vi "COM_MA filter.vi"(6 "Fs":dbl, 8 "Error In":errorcluster, 10 "Data In":dbl[](array[numeric])) -> (0 "Error Out":errorcluster, 2 "Data Out":dbl[](array[numeric]))   [LabVIEW 2017, in "AppPlugins.lvlib" / "EraPlugin.lvclass"]
uses:
  EraPlugin.lvclass
  <vilib>/Analysis/4window.llb/windowTd.ctl
  <vilib>/Analysis/3filter.llb/FIR Filter (DBL).vi
  <vilib>/Analysis/4window.llb/Symmetric Window (DBL).vi
  <vilib>/Analysis/NI_AALPro.lvlib
  <vilib>/Analysis/NI_AALBase.lvlib
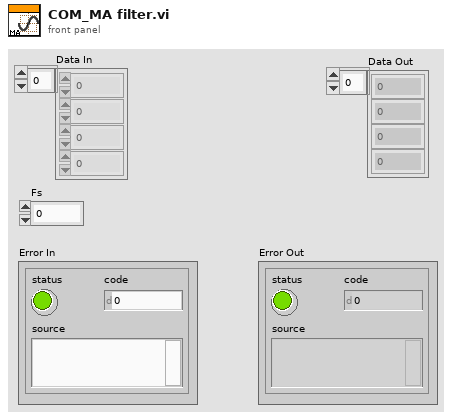
[diagram p1: front panel]
types:
  T1 = typedef "NI_AALPro.lvlib/windowTd.ctl" = u32
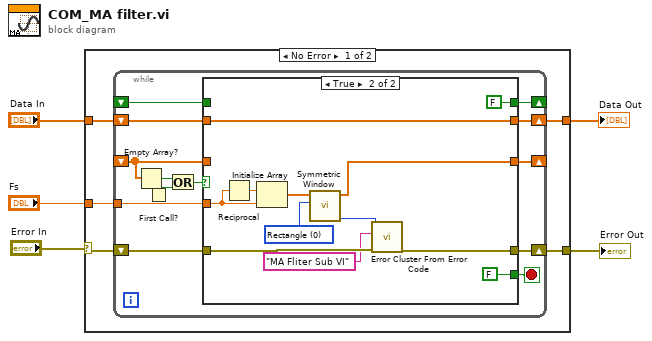
[diagram p0: block diagram]
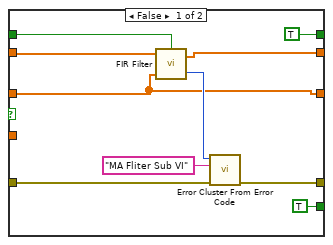
[diagram p2: hidden frame]
diagram:
  n1 = case shown="No Error" "Error In" {
    selector: "Error In" -> [w7 w46]
    tunnel: "Fs" -> [w10 _]
    tunnel: "Data In" -> [w9 _]
    tunnel: [w8 _] -> w3
    tunnel: [w6 w46] -> w1
    frame No Error {
      n2 = while {
        tunnel: w10 -> [w23]
        shift-right: [w21] -> w8
        shift-left: w9 -> [w22]
        shift-right: [w19] -> w6
        shift-left: w7 -> [w20]
        shift-right: [w15] -> _
        shift-left: _ -> [w14]
        shift-right: [w12] -> _
        shift-left: _ -> [w11]
        stop <- w18 stop-if-true
        n3 = Empty Array?(array=w14) -> (empty?=w16:bool)
        n4 = First Call?() -> (First Call?: T/F=w17:bool)
        n5 = Or(x=w16, y=w17) -> (x .or. y?=w13:bool)
        n6 = case shown="True" w13 {
          tunnel: w23 -> [_ w43]
          tunnel: w22 -> [w33 w37]
          tunnel: [w32 w37] -> w21
          tunnel: w20 -> [w31 w40]
          tunnel: [w30 w35] -> w19
          tunnel: [TRUE FALSE] -> w18
          tunnel: [w25 w36] -> w15
          tunnel: w14 -> [w25 _]
          tunnel: [TRUE ("init/cont (init:F)") FALSE ("init/cont (init:F)")] -> w12
          tunnel: w11 -> [w26 _]
          frame False {
            n7 = call-poly <vilib>:"FIR Filter.vi"("init/cont (init:F)"=w26, "FIR Coefficients"=w25, "X"=w33) -> ("error"=w28:i32, "Filtered X"=w32:dbl[])  [unwired: 1 in]
            n8 = call <vilib>:"Error Cluster From Error Code.vi"("error in (no error)"=w31, "error message (\"\")"="MA Fliter Sub VI" ("error message (\"\")"), "error code (0)"=w28) -> ("error out"=w30:errorcluster)  [unwired: 6 in]
          }
          frame True {
            w45 = T1 0 items=["Rectangle"=0, "Hanning"=1, "Hamming"=2, "Blackman-Harris"=3, "Exact Blackman"=4, "Blackman"=5, "Flat Top"=6, "4 Term B-Harris "=7, "7 Term B-Harris"=8, "Low Sidelobe"=9, "Blackman Nuttall"=11, "Triangle"=30, "Bartlett-Hanning"=31, "Bohman"=32, "Parzen"=33, "Welch"=34, "Kaiser"=60, "Dolph-Chebyshev"=61, "Gaussian"=62] ("window")
            n9 = Reciprocal(x=w43) -> (1/x=w42:dbl)
            n10 = Initialize Array(w42, w43) -> (w44:dbl[])
            n11 = call-poly <vilib>:"Symmetric Window.vi"("window"=w45, "X"=w44) -> ("error"=w41:i32, "Windowed X"=w36:dbl[])  [unwired: 1 in, 7 out]
            n12 = call <vilib>:"Error Cluster From Error Code.vi"("error in (no error)"=w40, "error message (\"\")"="MA Fliter Sub VI" ("error message (\"\")"), "error code (0)"=w41) -> ("error out"=w35:errorcluster)  [unwired: 6 in]
          }
        }
      }
    }
    frame Error {
    }
  }
  "Data Out" <- w3
  "Error Out" <- w1
